vi "Dashboard Main.vi"() -> ()   [LabVIEW 2017]
uses:
  <vilib>/Utility/miscctls.llb/LVRowAndColumnTypeDef.ctl
  <vilib>/event_ctls.llb/eventvkey.ctl
  <vilib>/Rock Robotics/Network Tables/NT Read Numeric Array.vi
  <vilib>/Rock Robotics/WPI/Dashboard/WPI_DashboardLogging Global.vi
panel:
  in  "Camera Settings Right":T1={"Frame Rate"=30, "Compression"=30, "Size"=1, "DB Camera Config"=FALSE} {"Frame Rate" scale=1.0..30.0; "Compression" scale=100.0..-1.0; "Size" items=["640x480", "320x240", "160x120"]}
  in  "Camera Name Right":string(combo)="No Camera Selection"
  out "Camera Info":cluster{"Mbps LED":bool, "Mbps":dbl, "fps":dbl} {"fps" format="%#.1g"; "Mbps" format="%#.1g"}
  in  "Camera Settings":T1={"Frame Rate"=30, "Compression"=30, "Size"=1, "DB Camera Config"=FALSE} {"Frame Rate" scale=1.0..30.0; "Compression" scale=100.0..-1.0; "Size" items=["640x480", "320x240", "160x120"]}
  in  "TCP":refnum<k5>
  in  "Rec Mode":enum32{"Stop", "Record", "Playback"}(radio)
  out "Robot IP":string
  out "Image Message":string="Timeout in Camera Communications"
  in  "Dashboard Tab":T2(tab)
  in  "Select Auto":string(combo)="Select Autonomous ..."
  out "NT Connection":bool
  out "MotorChart R":cluster{"Numeric":dbl, "Numeric":dbl}(graph)
  out "MotorChart L":cluster{"Numeric":dbl, "Numeric":dbl}(graph)
  out "MotorSliders R":cluster{"MotorSlide1":dbl, "MotorSlide2":dbl} {"MotorSlide2" scale=-1.0..1.0 scale format="%#_2e"; "MotorSlide1" scale=-1.0..1.0 scale format="%#_2e"}
  out "MotorSliders L":cluster{"MotorSlide1":dbl, "MotorSlide2":dbl} {"MotorSlide2" scale=-1.0..1.0 scale format="%#_2e"; "MotorSlide1" scale=-1.0..1.0 scale format="%#_2e"}
  out "Gyro":dbl(knob) scale=0.0..360.0
  out "JS1 Z":dbl(slide) scale=-1.0..1.0 scale format="%#_2e"
  out "JS1 Graph":cluster{"X":dbl, "Y":dbl}[](graph)
  out "JS1 Buttons":T3
  out "JS2 Z":dbl(slide) scale=-1.0..1.0 scale format="%#_2e"
  out "JS2 Graph":cluster{"X":dbl, "Y":dbl}[](graph)
  out "JS2 Buttons":T3
  out "Mode":T4(ring)=enum."Auto Disabled"
  out "Camera Image Right":T5(plugin-control)
  in  "DB/String 9":string
  in  "DB/String 8":string
  in  "DB/String 7":string
  in  "DB/String 6":string
  in  "DB/String 5":string
  in  "DB/String 4":string
  in  "DB/String 3":string
  in  "DB/String 2":string
  in  "DB/String 1":string
  in  "DB/String 0":string
  in  "DB/Slider 0":dbl(slide) scale=0.0..5.0
  in  "DB/Slider 1":dbl(slide) scale=0.0..5.0
  in  "DB/Slider 2":dbl(slide) scale=0.0..5.0
  in  "DB/Slider 3":dbl(slide) scale=0.0..5.0
  out "DB/LED 3":bool
  out "DB/LED 2":bool
  out "DB/LED 1":bool
  out "DB/LED 0":bool
  in  "DB/Button 3":bool
  in  "DB/Button 2":bool
  in  "DB/Button 1":bool
  in  "DB/Button 0":bool caption="New Name"
  in  "When Switch on Same Side\nAnd Scale on Wrong Side":u16(ring) items=["Do Nothing"=0, "Cross Auto Line"=4]
  in  "When Switch on Opposite Side\nAnd Scale on Wrong Side":u16(ring) items=["Do Nothing"=0, "Cross AutoLine"=4]
  in  "Direction":u16(ring) items=["Forward (Cube in forks)", "Backward (Cube on shelf)"]
  in  "Starting Position":u16(ring) items=["Left", "Center-Left", "Center", "Center-Right", "Right"]
  in  "When Switch on Opposite Side":u16(ring) items=["Do Nothing"=0, "Cross in Front"=1, "Cross Behind"=2, "Cross Auto Line"=4, "Drive to Null Territory"=5, "Check Scale"=3]
  in  "When Switch on Same Side":u16(ring) items=["Do Nothing"=0, "Proceed"=1, "Drive to Null Territory"=5, "Cross Auto Line"=4, "Check Scale"=3]
  in  "When Switch on Right Side":u16(ring) items=["Do Nothing", "Proceed"]
  in  "When Switch on Left SIde":u16(ring) items=["Do Nothing", "Proceed"]
  in  "Test Slider":dbl(slide) scale=0.0..100.0 scale format="%#_3g"
  in  "On/Off":bool caption="Solenoid"
  in  "Test Name":u16(ring) items=["Select the test to run..."]
  in  "Test Tree":string(tree)
  in  "Motor":cluster{"Value":dbl, "Enable":bool} {"Value" scale=-1.0..1.0 scale format="%#_3g"}
  out "Progress":T6 {"Test Progress" scale=0.0..100.0}
  in  "Rev/Fwd":cluster{"Forward":bool, "Reverse":bool}
  in  "Test Ring":u16(ring) items=["Monochrome", "Color"]
  out "Cmd Status":string
  in  "Execute Command":bool
  in  "Command Params":string[][](table)
  in  "Command Selection":i32(listbox)
  in  "CheckList":i32(listbox)
  out "Tree":string(tree)
  out "Camera Image":T5(plugin-control)
  out "Background":bool
  in  "Camera Name":string(combo)="No Camera Selection"
  # "HW"
  # "HW"
  # "Joysticks"
  # "Drive Motors"
  # "Front"
  # "Right"
  # "Left"
  # "Back"
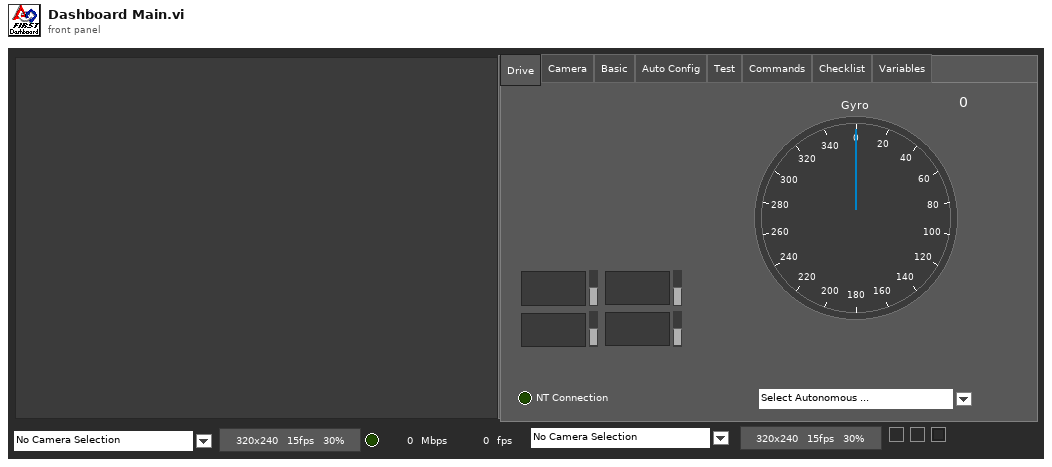
[diagram p1: front panel]
types:
  T1 = cluster{"Frame Rate":i32, "Compression":i32, "Size":u16, "DB Camera Config":bool}
  T2 = enum32{"Drive", "Camera", "Basic", "Auto Config", "Test", "Commands", "Checklist", "Variables"}
  T3 = cluster{bool, bool, bool, bool, bool, bool, bool, bool, bool, bool, bool, bool}
  T4 = enum8{"Tele-Op Disabled", "Tele-Op Enabled", "Auto Disabled", "Auto Enabled", "Test Disabled", "Test Enabled", "Disconnected", "No Code", "E-Stop"}
  T5 = typedef "IMAQ Image.ctl" = refnum<image>
  T6 = cluster{"Test Progress":u8, "Test Progress Text":string}
  T7 = cluster{"Save Path":path, "Interval (s)":dbl, "Keep":i32}
  T8 = enum32{"Drive", "Camera", "Basic", "Custom", "Test", "Commands", "Checklist", "Variables"}
  T9 = typedef "Image Type" = u32
  T10 = cluster{"IDs":cluster{"RPC field ID":u16, "Unique ID":u16}, "String":string}
  T11 = cluster{"Error Strings":string, "Disable Counts":cluster{u16, u16}, "Rail Faults":cluster{u16, u16, u16}, "Robot IP":string, "DB Mode":u8, "Event Info":cluster{"Name":string, "Type":u8, "Number":u16, "Replay":u8}}
  T12 = cluster{"Storage":cluster{"Disk Free":u64, "RAM Block":u32, "RAM free":u32}, "CPU Utilization":cluster{"CPU % ISR":sgl, "CPU % Time Crit":sgl, "CPU % Timed Str":sgl, "CPU % High":sgl, "CPU % Above":sgl, "CPU % Normal":sgl, "CPU % Low":sgl}, "CAN":cluster{"% Bus Utilization":sgl, "Bus Off Cnt":u32, "TX_FIFO Full Cnt":u32, "Receive Error Cnt":u8, "Transmit Error Cnt":u8}, "HID":cluster{"HID Outputs":u32, "Rumble Low":u16, "Rumble High":u16}[]}
  T13 = cluster{"Status bits":cluster{"Test Mode":bool, "Autonomous":bool, "Enabled":bool, "Code Start":bool, "Brownout":bool, "Reserved 2":bool, "Reserved 3":bool, "E-Stop":bool}, "Code Trace":cluster{"Disabled":bool, "TeleOp":bool, "Auto":bool, "Test":bool}, "Controller Type":enum16{"unknown", "cRIO", "roboRio"}, "Code?":enum16{"unknown", "noCode", "code"}, "Battery V":dbl}
  T14 = cluster{"Control Bits":cluster{"TestMode":bool, "Autonomous":bool, "Enabled":bool, "FMS Present":bool, bool, bool, bool, "E-Stop":bool}, "Team Station ":u8, "Countdown":sgl, "Joystick Values":cluster{"Axes":dbl[], "Buttons":bool[], "POVs":i16[]}[]}
  T15 = cluster{"Axes":dbl[], "Buttons":bool[], "POVs":i16[]}[]
  T16 = cluster{"Axes":dbl[], "Buttons":bool[], "POVs":i16[]}
  T17 = cluster{"Buttons[0]":bool, "Buttons[1]":bool, "Buttons[2]":bool, "Buttons[3]":bool, "Buttons[4]":bool, "Buttons[5]":bool, "Buttons[6]":bool, "Buttons[7]":bool, "Buttons[8]":bool, "Buttons[9]":bool, "Buttons[10]":bool, "Buttons[11]":bool}
  T18 = cluster{"Camera Image":refnum<vi>, "Dashboard Tab":refnum<vi>, "Background":refnum<vi>, "Rec Mode":refnum<vi>, "Test Slider":refnum<vi>, "On/Off ":refnum<vi>, "Test Ring":refnum<vi>, "Rev/Fwd":refnum<vi>, "Test Name":refnum<vi>, "Motor":refnum<vi>, "Progress":refnum<vi>, "CheckList":refnum<vi>, "Tree":refnum<vi>, "Test Tree":refnum<vi>, "Command Params":refnum<vi>, "Command Selection":refnum<vi>, "Execute Command":refnum<vi>, "Cmd Status":refnum<vi>, "Camera Settings":refnum<vi>, "Camera Name":refnum<vi>, "Camera Info":refnum<vi>, "Camera Settings Right":refnum<vi>, "Camera Name Right":refnum<vi>, "Camera Image Right":refnum<vi>}
  T19 = cluster{"Camera Name Right":string, string, "Saved DB Images Info":cluster{"Save Path":path, "Interval (s)":dbl, "Keep":i32}}
  T20 = cluster{"Camera Name":string, string, "Saved DB Images Info":cluster{"Save Path":path, "Interval (s)":dbl, "Keep":i32}}
  T21 = cluster{"Operation":enum16{"Update", "Clear"}, "Color Box":u32}[]
  T22 = typedef "eventvkey.ctl" = enum16{"ASCII", "Enter", "Return", "Shift", "Ctrl", "Alt", "Cmd", "Opt", "Caps", "NumLock", "Clear", "Break", "Up", "Down", "Left", "Right", "Insert", "Delete", "Home", "End", "PageUp", "PageDown", "Escape", "Help", "Pause", "ScrollLock", "F1", "F2", "F3", "F4", "F5", "F6", "F7", "F8", "F9", "F10", "F11", "F12", "F13", "F14", "F15", "F16", "F17", "F18", "F19", "F20", "F21", "F22", "F23", "F24", "Play", "VolumeUp", "VolumeDown", "Mute", "Two Byte Char"}
  T23 = cluster{"Image Size":bool, "Image Type":bool, "Pixel Value":bool, "ROI Information":bool, "Zoom Factor":bool}
  T24 = cluster{"Operation":enum16{"Update", "Clear"}, "Color Box":u32}
  T25 = typedef "LVRowAndColumnTypeDef.ctl" = cluster{"Row":i32, "Column":i32}
  T26 = cluster{"Shift":bool, "Ctrl":bool, "Alt":bool, "Cmd":bool, "Opt":bool}
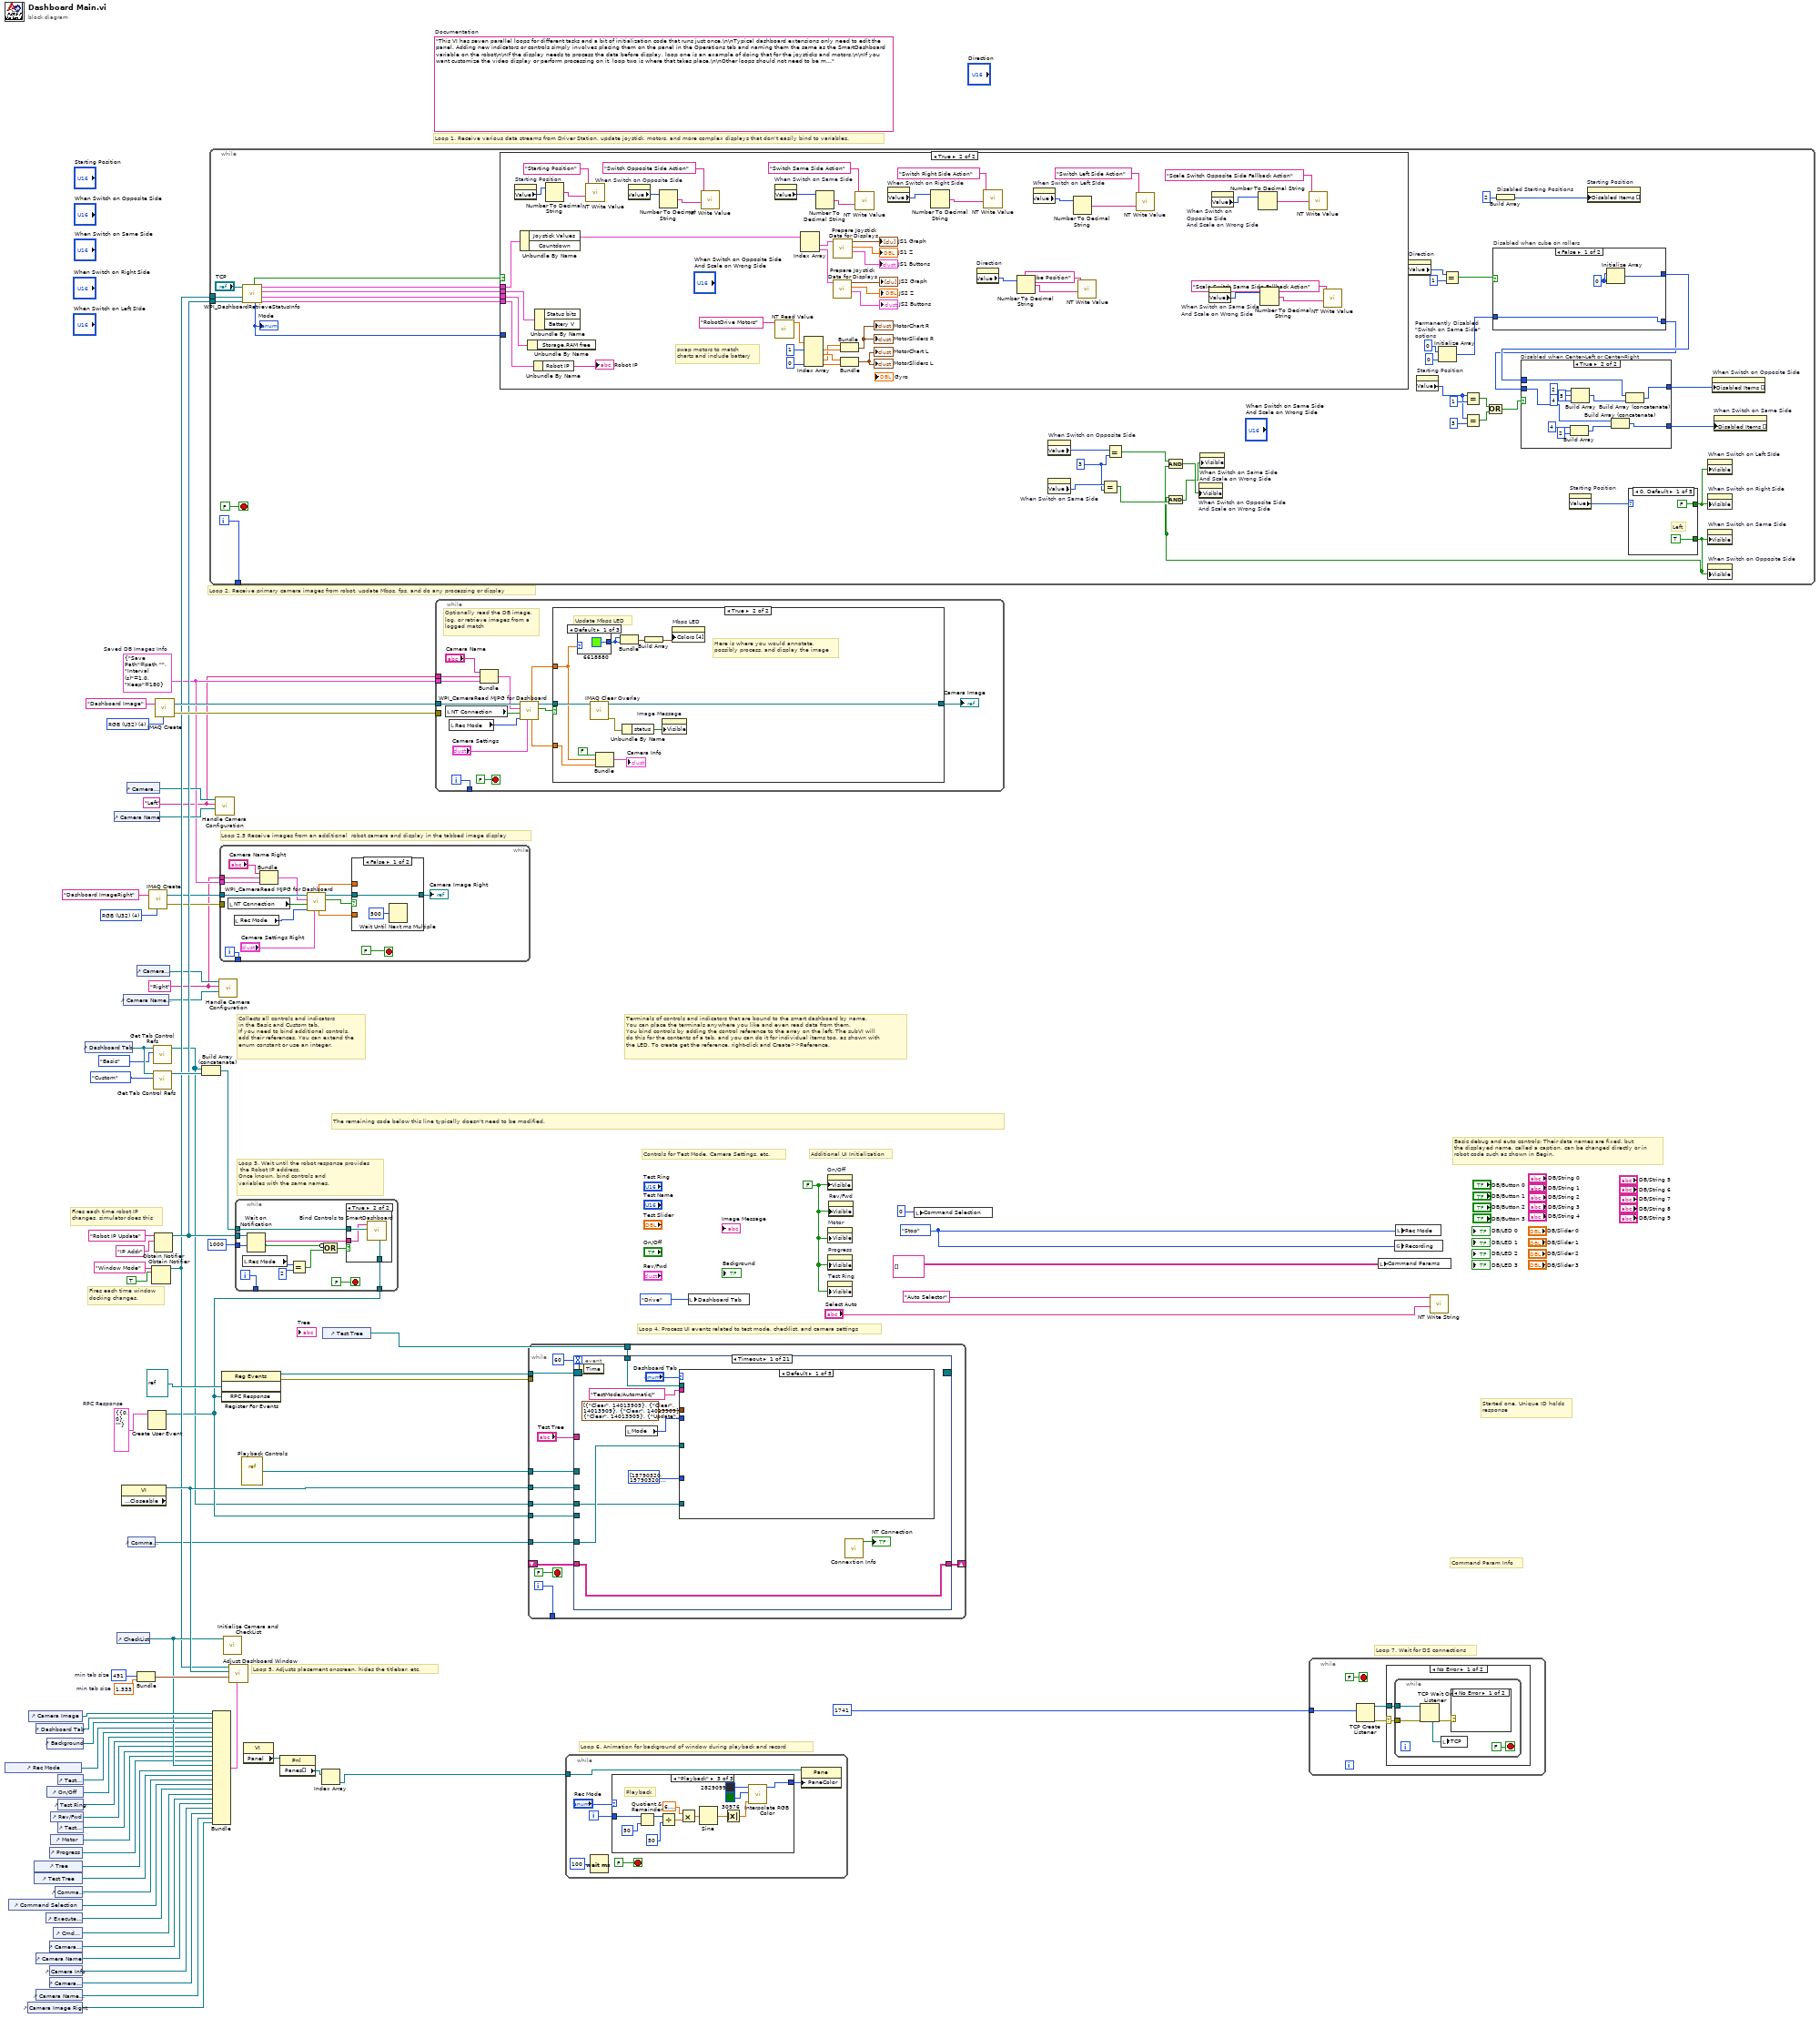
[diagram p0: block diagram]
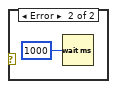
[diagram p3: hidden frame]
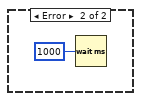
[diagram p4: hidden frame]
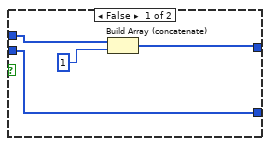
[diagram p5: hidden frame]
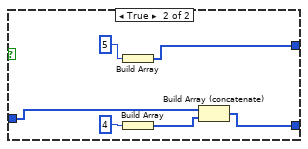
[diagram p6: hidden frame]
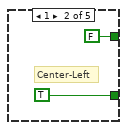
[diagram p7: hidden frame]
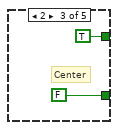
[diagram p8: hidden frame]
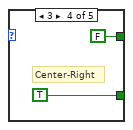
[diagram p9: hidden frame]
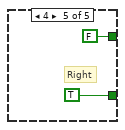
[diagram p10: hidden frame]
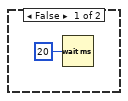
[diagram p11: hidden frame]
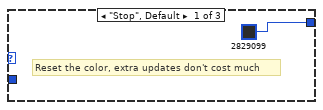
[diagram p12: hidden frame]
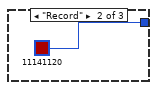
[diagram p13: hidden frame]
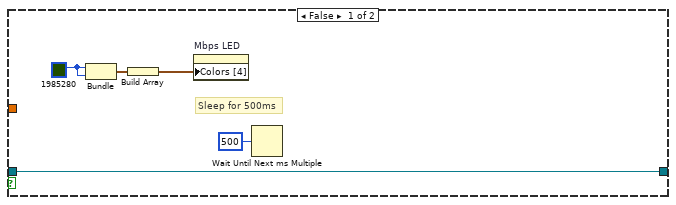
[diagram p15: hidden frame]
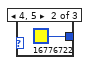
[diagram p16: hidden frame]
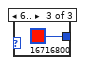
[diagram p17: hidden frame]
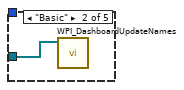
[diagram p18: hidden frame]
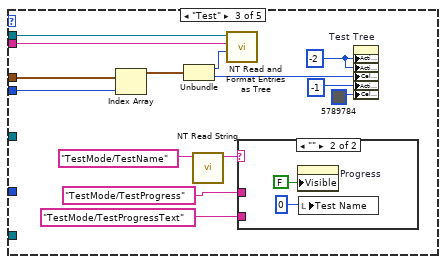
[diagram p19: hidden frame]
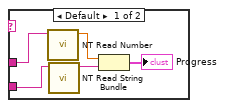
[diagram p20: hidden frame]
diagram:
  w3 = T7 {"Save Path"=path "", "Interval (s)"=1.0, "Keep"=180}  # Saved DB Images Info
  w2 = "Right"
  w1 = "Left"
  w13 = T9 4 items=["Grayscale (U8)", "Grayscale (I16)", "Grayscale (SGL)", "Complex (CSG)", "RGB (U32)", "HSL (U32)", "RGB (U64)"] ("Image Type")
  w29 = T10 {"IDs"={"RPC field ID"=0, "Unique ID"=0}, "String"=""}  # RPC Response
  w52 = 491  # min tab size
  w51 = 1.333  # min tab size
  w59 = enum32{"Stop", "Record", "Playback"}."Stop" ("Rec Mode")
  w36 = FALSE ("Visible")
  (unwired) "This VI has seven parallel loops for different tasks and a bit of initialization code that runs just once.\n\nTypical dashboard extensions only need to edit the panel. Adding new indicators or controls simply involves placing them on the panel in the Operations tab and naming them the same as the SmartDashboard variable on the robot\n\nIf the display needs to process the data before display, loop one is an example of doing that for the joysticks and motors.\n\nIf you want customize the video display or perform processing on it, loop two is where that takes place.\n\nOther loops should not need to be modified. They are pretty standard, and document the task they perform."  # Documentation
  w76 = T9 4 items=["Grayscale (U8)", "Grayscale (I16)", "Grayscale (SGL)", "Complex (CSG)", "RGB (U32)", "HSL (U32)", "RGB (U64)"] ("Image Type")
  # "Loop 2.5 Receive images from an additional  robot camera and display in the tabbed image display"
  # "Command Param Info"
  # "Started one, Unique ID holds\nresponse"
  # "Loop 7. Wait for DS connections"
  # "Basic debug and auto controls: Their data names are fixed, but\nthe displayed name, called a caption, can be changed directly or in\nrobot code such as shown in Begin."
  # "Controls for Test Mode, Camera Settings, etc."
  # "Additional UI Initialization"
  # "Loop 6. Animation for background of window during playback and record"
  # "Fires each time robot IP\nchanges, simulator does this"
  # "Fires each time window\ndocking changes."
  # "Collects all controls and indicators\nin the Basic and Custom tab.\nIf you need to bind additional controls,\nadd their references. You can extend the\nenum constant or use an integer."
  # "The remaining code below this line typically doesn't need to be modified."
  # "Loop 4. Process UI events related to test mode, checklist, and camera settings"
  # "Terminals of controls and indicators that are bound to the smart dashboard by name.\nYou can place the terminals anywhere you like and even read data from them.\nYou bind controls by adding the control reference to the array on the left. The subVI will\ndo this for the contents of a tab, and you can do it for individual items too, as shown with\nthe LED. To create get the reference, right-click and Create>>Reference."
  # "Loop 3. Wait until the robot response provides\n the Robot IP address.\nOnce known, bind controls and\nvariables with the same names."
  # "Loop 5. Adjusts placement onscreen, hides the titlebar, etc."
  # "Loop 1. Receive various data streams from Driver Station, update joystick, motors, and more complex displays that don't easily bind to variables."
  # "Loop 2. Receive primary camera images from robot, update Mbps, fps, and do any processing or display"
  n1 = control-ref of="Rec Mode"() -> (w42:refnum<vi>)
  n2 = control-ref of="Command Selection"() -> (w28:refnum<vi>)
  n3 = control-ref of="Camera Image Right"() -> (w6:refnum<vi>)
  n4 = control-ref of="Camera Image"() -> (w54:refnum<vi>)
  n5 = control-ref of="Tree"() -> (w46:refnum<vi>)
  n6 = control-ref of="Test Tree"() -> (w45:refnum<vi>)
  n7 = control-ref of="Dashboard Tab"() -> (w53:refnum<vi>)
  n8 = control-ref of="Camera Name"() -> (w19:refnum<vi>)
  n9 = control-ref of="Camera Name Right"() -> (w7:refnum<vi>)
  n10 = control-ref of="Execute Command"() -> (w30:refnum<vi>)
  n11 = control-ref of="Background"() -> (w49:refnum<vi>)
  n12 = control-ref of="On/Off"() -> (w40:refnum<vi>)
  n13 = control-ref of="Progress"() -> (w37:refnum<vi>)
  n14 = control-ref of="Camera Settings"() -> (w20:refnum<vi>)
  n15 = control-ref of="Camera Info"() -> (w18:refnum<vi>)
  n16 = control-ref of="Camera Settings Right"() -> (w8:refnum<vi>)
  n17 = control-ref of="Rev/Fwd"() -> (w38:refnum<vi>)
  n18 = control-ref of="Motor"() -> (w43:refnum<vi>)
  n19 = control-ref of="Cmd Status"() -> (w24:refnum<vi>)
  n20 = control-ref of="Command Params"() -> (w31:refnum<vi>)
  n21 = control-ref of="Test Slider"() -> (w41:refnum<vi>)
  n22 = control-ref of="Test Ring"() -> (w39:refnum<vi>)
  n23 = control-ref of="Test Name"() -> (w44:refnum<vi>)
  n24 = control-ref of="Dashboard Tab"() -> (w57:refnum<vi>)
  n25 = control-ref of="Camera Name"() -> (w21:refnum<vi>)
  n26 = control-ref of="CheckList"() -> (w47:refnum<vi>)
  n27 = property class="VI" props=["Front Panel.Closeable"]() -> (reference out=w58:refnum<vi>)  [unwired: 2 in, 2 out]
  n28 = control-ref of="Camera Name Right"() -> (w9:refnum<vi>)
  n29 = control-ref of="Camera Settings"() -> (w22:refnum<vi>)
  n30 = control-ref of="Command Params"() -> (w23:refnum<vi>)
  n31 = control-ref of="Camera Settings Right"() -> (w10:refnum<vi>)
  n32 = Bundle("min tab size"=w52, "min tab size"=w51) -> (w50:cluster{"min tab size":i32, "min tab size":dbl})  [unwired: 1 in]
  n33 = Create User Event(user event datatype=w29) -> (user event=w25:refnum<user-event>)  [unwired: 1 in, 1 out]
  n34 = call "IMAQ Create"("Image Name"="Dashboard ImageRight", "Image Type"=w13) -> ("New Image"=w12:T5, "error out"=w11:errorcluster)  [unwired: 2 in, 1 out]
  n35 = Obtain Notifier(name (unnamed)="Window Mode", notification data type=TRUE) -> (notifier out=w34:refnum<notifier>)  [unwired: 2 in, 2 out]
  n36 = call <vilib>:"Get Tab Control Refs.vi"("Page Index"=T8."Basic" ("Dashboard Tab"), "TabControl in"=w57) -> ("ControlsOnPage"=w17:refnum<vi>[])  [unwired: 9 in]
  n37 = call <vilib>:"Get Tab Control Refs.vi"("Page Index"=T8."Custom" ("Dashboard Tab"), "TabControl in"=w57) -> ("ControlsOnPage"=w56:refnum<vi>[])  [unwired: 9 in]
  n38 = Obtain Notifier(name (unnamed)="Robot IP Update", notification data type="IP Addr" ("name (unnamed)")) -> (notifier out=w35:refnum<notifier>)  [unwired: 2 in, 2 out]
  n39 = call "IMAQ Create"("Image Name"="Dashboard Image", "Image Type"=w76) -> ("New Image"=w74:T5, "error out"=w73:errorcluster)  [unwired: 2 in, 1 out]
  n40 = Build Array (concatenate)(w17, w56) -> (w55:refnum<vi>[])
  n41 = while {
    tunnel: [w114] -> _
    tunnel: w35 -> [w108]
    tunnel: w34 -> [w105]
    i -> [w114]
    stop <- FALSE stop-if-true
    w82 = 3
    n42 = call <vilib>:"WPI_DashboardRetrieveStatusInfo.vi"("Binding Refnum"=w108, "Window Mode Notifier"=w105, "TCP Cnx"="TCP") -> ("Power and Errors"=w109:T11, "Robot Metrics"=w112:T12, "Status Info"=w113:T13, "Control Info"=w110:T14, "Robot Mode"=w107:T4, "Process?"=w111:bool)  [unwired: 3 in]
    "Mode" <- w107
    n43 = case shown="True" w111 {
      tunnel: w113 -> [_ w198]
      tunnel: w112 -> [_ w197]
      tunnel: w110 -> [_ w196]
      tunnel: w109 -> [_ w195]
      tunnel: w107 -> [_ _]
      frame False {
        n44 = Wait (ms)(milliseconds to wait=u32 20) -> ()  [unwired: 1 out]
      }
      frame True {
        # "swap motors to match\ncharts and include battery"
        n45 = property on="Starting Position" class="Ring (strict)"() -> ("Value"=w172:u16)  [unwired: 2 in, 2 out]
        n46 = Unbundle By Name(w196) -> ("Joystick Values"=w186:T15)  [unwired: 1 out]
        n47 = Unbundle By Name(w197) -> ()  [unwired: 1 out]
        n48 = Unbundle By Name(w195) -> ("Robot IP"=→"Robot IP":string)
        n49 = Unbundle By Name(w198) -> ()  [unwired: 2 out]
        n50 = Number To Decimal String(number=w172) -> (decimal integer string=w174:string)  [unwired: 1 in]
        n51 = call-poly <vilib>:"NT Write Value.vi"("String"=w174, "Name"="Starting Position") -> ()  [unwired: 9 in, 1 out]
        n52 = property on="When Switch on Opposite Side" class="Ring (strict)"() -> ("Value"=w171:u16)  [unwired: 2 in, 2 out]
        n53 = Number To Decimal String(number=w171) -> (decimal integer string=w157:string)  [unwired: 1 in]
        n54 = call-poly <vilib>:"NT Write Value.vi"("String"=w157, "Name"="Switch Opposite Side Action") -> ()  [unwired: 9 in, 1 out]
        n55 = property on="When Switch on Same Side" class="Ring (strict)"() -> ("Value"=w170:u16)  [unwired: 2 in, 2 out]
        n56 = call-poly <vilib>:"NT Read Value.vi"("Name"="RobotDrive Motors") -> ("Numeric Array"=w176:dbl[])  [unwired: 9 in, 1 out]
        n57 = Index Array(array=w186) -> (element #1=w185:T16, element #2=w181:T16)  [unwired: 2 in]
        n58 = Index Array(array=w176, index #1=1, index #4=0) -> (element #1=w190:dbl, element #2=w191:dbl, element #3=w189:dbl, element #4=w194:dbl)  [unwired: 2 in]
        n59 = Number To Decimal String(number=w170) -> (decimal integer string=w167:string)  [unwired: 1 in]
        n60 = call "Prepare Joystick Data for Displays.vi"("Joystick Values"=w181) -> ("Buttons"=→"JS2 Buttons":T17, "Z Axis"=→"JS2 Z":dbl, "Cartesian Data"=→"JS2 Graph":cluster{"X axis":dbl, "X axis":dbl}[])  [unwired: 8 in]
        n61 = call "Prepare Joystick Data for Displays.vi"("Joystick Values"=w185) -> ("Buttons"=→"JS1 Buttons":T17, "Z Axis"=→"JS1 Z":dbl, "Cartesian Data"=→"JS1 Graph":cluster{"X axis":dbl, "X axis":dbl}[])  [unwired: 8 in]
        n62 = Bundle("Numeric"=w189, "Numeric"=w190) -> (→"MotorChart R" →"MotorSliders R":cluster{"Numeric":dbl, "Numeric":dbl})  [unwired: 1 in]
        n63 = Bundle("Numeric"=w191, "Numeric"=w194) -> (→"MotorChart L" →"MotorSliders L":cluster{"Numeric":dbl, "Numeric":dbl})  [unwired: 1 in]
        n64 = call-poly <vilib>:"NT Write Value.vi"("String"=w167, "Name"="Switch Same Side Action") -> ()  [unwired: 9 in, 1 out]
        n65 = property on="When Switch on Right Side" class="Ring (strict)"() -> ("Value"=w169:u16)  [unwired: 2 in, 2 out]
        n66 = Number To Decimal String(number=w169) -> (decimal integer string=w166:string)  [unwired: 1 in]
        n67 = property on="Direction" class="Ring (strict)"() -> ("Value"=w160:u16)  [unwired: 2 in, 2 out]
        n68 = call-poly <vilib>:"NT Write Value.vi"("String"=w166, "Name"="Switch Right Side Action") -> ()  [unwired: 9 in, 1 out]
        n69 = Number To Decimal String(number=w160) -> (decimal integer string=w159:string)  [unwired: 1 in]
        n70 = property on="When Switch on Left SIde" class="Ring (strict)"() -> ("Value"=w168:u16)  [unwired: 2 in, 2 out]
        n71 = Number To Decimal String(number=w168) -> (decimal integer string=w165:string)  [unwired: 1 in]
        n72 = call-poly <vilib>:"NT Write Value.vi"("String"=w159, "Name"="Cube Position") -> ()  [unwired: 9 in, 1 out]
        n73 = call-poly <vilib>:"NT Write Value.vi"("String"=w165, "Name"="Switch Left Side Action") -> ()  [unwired: 9 in, 1 out]
        n74 = property on="When Switch on Same Side\nAnd Scale on Wrong Side" class="Ring (strict)"() -> ("Value"=w153:u16)  [unwired: 2 in, 2 out]
        n75 = property on="When Switch on Opposite Side\nAnd Scale on Wrong Side" class="Ring (strict)"() -> ("Value"=w156:u16)  [unwired: 2 in, 2 out]
        n76 = Number To Decimal String(number=w156) -> (decimal integer string=w155:string)  [unwired: 1 in]
        n77 = Number To Decimal String(number=w153) -> (decimal integer string=w152:string)  [unwired: 1 in]
        n78 = call-poly <vilib>:"NT Write Value.vi"("String"=w155, "Name"="Scale Switch Opposite Side Fallback Action") -> ()  [unwired: 9 in, 1 out]
        n79 = call-poly <vilib>:"NT Write Value.vi"("String"=w152, "Name"="Scale Switch Same Side Fallback Action") -> ()  [unwired: 9 in, 1 out]
      }
    }
    n80 = property on="When Switch on Opposite Side" class="Ring (strict)"() -> ("Value"=w84:u16)  [unwired: 2 in, 2 out]
    n81 = property on="When Switch on Same Side" class="Ring (strict)"() -> ("Value"=w83:u16)  [unwired: 2 in, 2 out]
    n82 = Equal?(x=w83, y=w82) -> (x = y?=w80:bool)
    n83 = Equal?(x=w84, y=w82) -> (x = y?=w81:bool)
    n84 = property on="Direction" class="Ring (strict)"() -> ("Value"=w103:u16)  [unwired: 2 in, 2 out]
    n85 = property on="Starting Position" class="Ring (strict)"() -> ("Value"=w93:u16)  [unwired: 2 in, 2 out]
    n86 = Initialize Array "Permanently Disabled \"Switch on Same Side\" options"(0, 0 ("dimension size")) -> (w97:i32[])
    n87 = Equal?(x=w103, y=u16 1) -> (x = y?=w101:bool)
    n88 = Equal?(x=w93, y=u16 1) -> (x = y?=w89:bool)
    n89 = Equal?(x=w93, y=u16 3) -> (x = y?=w91:bool)
    n90 = Or(x=w89, y=w91) -> (x .or. y?=w90:bool)
    n91 = case "Disabled when cube on rollers" shown="False" w101 {
      tunnel: [w132 w134] -> w88
      tunnel: [w133 w135] -> w86
      tunnel: w97 -> [w133 w137]
      frame False {
        w131 = 0 ("dimension size")
        n92 = Initialize Array(w131, w131) -> (w132:i32[])
      }
      frame True {
        n93 = Build Array(5) -> (w134:i32[])
        n94 = Build Array(4) -> (w136:i32[])
        n95 = Build Array (concatenate)(w137, w136) -> (w135:i32[])
      }
    }
    n96 = Build Array "Disabled Starting Positions"(2) -> (w98:i32[])
    n97 = case "Disabled when Center-Left or Center-Right" shown="True" w90 {
      tunnel: w88 -> [w118 w127]
      tunnel: [w117 w126] -> w87
      tunnel: w86 -> [w119 w123]
      tunnel: [w119 w122] -> w85
      frame False {
        n98 = Build Array (concatenate)(w118, 1) -> (w117:i32[])
      }
      frame True {
        n99 = Build Array(4, 2 ("element")) -> (w124:i32[])
        n100 = Build Array(2, 5 ("element"), 4 ("element")) -> (w128:i32[])
        n101 = Build Array (concatenate)(w123, w124) -> (w122:i32[])
        n102 = Build Array (concatenate)(w127, w128) -> (w126:i32[])
      }
    }
    n103 = property on="Starting Position" class="Ring (strict)"() -> ("Value"=w100:u16)  [unwired: 2 in, 2 out]
    n104 = property on="Starting Position" class="Ring (strict)"("Disabled Items []"=w98) -> ()  [unwired: 2 in, 2 out]
    n105 = case shown="0, Default" w100 {
      tunnel: [TRUE TRUE FALSE TRUE TRUE] -> w79
      tunnel: [FALSE FALSE TRUE FALSE FALSE] -> w104
      frame 0, Default {
        # "Left"
      }
      frame 1 {
        # "Center-Left"
      }
      frame 2 {
        # "Center"
      }
      frame 3 {
        # "Center-Right"
      }
      frame 4 {
        # "Right"
      }
    }
    n106 = And(x=w81, y=w79) -> (x .and. y?=w78:bool)
    n107 = And(x=w79, y=w80) -> (x .and. y?=w77:bool)
    n108 = property on="When Switch on Opposite Side\nAnd Scale on Wrong Side" class="Ring (strict)"("Visible"=w78) -> ()  [unwired: 2 in, 2 out]
    n109 = property on="When Switch on Same Side\nAnd Scale on Wrong Side" class="Ring (strict)"("Visible"=w77) -> ()  [unwired: 2 in, 2 out]
    n110 = property on="When Switch on Left SIde" class="Ring (strict)"("Visible"=w104) -> ()  [unwired: 2 in, 2 out]
    n111 = property on="When Switch on Right Side" class="Ring (strict)"("Visible"=w104) -> ()  [unwired: 2 in, 2 out]
    n112 = property on="When Switch on Same Side" class="Ring (strict)"("Visible"=w79) -> ()  [unwired: 2 in, 2 out]
    n113 = property on="When Switch on Opposite Side" class="Ring (strict)"("Visible"=w79) -> ()  [unwired: 2 in, 2 out]
    n114 = property on="When Switch on Opposite Side" class="Ring (strict)"("Disabled Items []"=w87) -> ()  [unwired: 2 in, 2 out]
    n115 = property on="When Switch on Same Side" class="Ring (strict)"("Disabled Items []"=w85) -> ()  [unwired: 2 in, 2 out]
  }
  n116 = Bundle("Camera Image"=w54, "Dashboard Tab"=w53, "Background"=w49, "Rec Mode"=w42, "Test Slider"=w41, "On/Off"=w40, "Test Ring"=w39, "Rev/Fwd"=w38, "Test Name"=w44, "Motor"=w43, "Progress"=w37, "CheckList"=w47, "Tree"=w46, "Test Tree"=w45, "Command Params"=w31, "Command Selection"=w28, "Execute Command"=w30, "Cmd Status"=w24, "Camera Settings"=w20, "Camera Name"=w19, "Camera Info"=w18, "Camera Settings Right"=w8, "Camera Name Right"=w7, "Camera Image Right"=w6) -> (w48:T18)  [unwired: 1 in]
  n117 = call "Handle Camera Configuration.vi"("CameraNameRef"=w21, "Display Name"=w1, "ClusterRef"=w22) -> ()  [unwired: 9 in]
  n118 = call "Handle Camera Configuration.vi"("CameraNameRef"=w9, "Display Name"=w2, "ClusterRef"=w10) -> ()  [unwired: 9 in]
  n119 = while {
    tunnel: w12 -> [w213]
    tunnel: w11 -> [_]
    tunnel: [w208] -> _
    tunnel: w3 -> [w202]
    tunnel: w2 -> [w199]
    i -> [w208]
    stop <- FALSE stop-if-true
    n120 = local read "NT Connection"() -> (w203:bool)
    n121 = local read "Rec Mode"() -> (w212:enum32{"Stop", "Record", "Playback"})
    n122 = Bundle("Camera Name Right"="Camera Name Right", w199, "Saved DB Images Info"=w202) -> (w201:T19)  [unwired: 1 in]
    n123 = call <vilib>:"WPI_CameraRead MJPG for Dashboard.vi"("Camera Settings"="Camera Settings Right", "Rec Mode"=w212, "NT Connection"=w203, "Capture Info"=w201, "Refnum in"=w213) -> ("Active"=w207:bool, "Refnum out"=w210:T5, "FPS"=w205:dbl, "Bandwidth (Mbps)"=w206:dbl)  [unwired: 3 in]
    n124 = case shown="False" w207 {
      tunnel: w210 -> [w214 w216]
      tunnel: w206 -> [_ _]
      tunnel: w205 -> [_ _]
      tunnel: [w214 w216] -> w204
      frame False {
        n125 = Wait Until Next ms Multiple(millisecond multiple=u32 500) -> ()  [unwired: 1 out]
      }
      frame True {
      }
    }
    "Camera Image Right" <- w204
  }
  n126 = register-events(refnum<vi> refnum, w25) -> (reference out=w63:refnum<event-registration>, error out=w62:errorcluster)  [unwired: 2 in]
  n127 = call "Initialize Camera and CheckList.vi"("ListBox in"=w47) -> ()  [unwired: 11 in]
  n128 = call "Adjust Dashboard Window.vi"("Sizing Refnums"=w48, "Size Constraints"=w50, "VI"=w58, "WIn Mode"=w34) -> ()  [unwired: 8 in]
  n129 = while {
    tunnel: w55 -> [w228]
    tunnel: w35 -> [w226]
    tunnel: [w224] -> _
    tunnel: u32 1000 ("milliseconds to wait") -> [w223]
    tunnel: w25 -> [w217]
    i -> [w224]
    stop <- FALSE stop-if-true
    n130 = local read "Rec Mode"() -> (w219:enum32{"Stop", "Record", "Playback"})
    n131 = Wait on Notification(notifier=w226, timeout in ms (-1)=w223) -> (notification=w225:string, timed out?=w221:bool)  [unwired: 2 in, 2 out]
    n132 = Equal?(x=w219, y=u16 2 ("Rec Mode")) -> (x = y?=w220:bool)
    n133 = Compound Arithmetic op=OR(invert w221, w220) -> (w222:bool)
    n134 = case shown="True" w222 {
      tunnel: w228 -> [_ w231]
      tunnel: w225 -> [_ w230]
      tunnel: w217 -> [_ w229]
      frame False {
      }
      frame True {
        n135 = call <vilib>:"Bind Controls to SmartDashboard.vi"("RPC ref"=w229, "Bound Control Refs"=w231, "Server IP Address"=w230) -> ()  [unwired: 9 in]
      }
    }
  }
  n136 = vi-ref "Playback Controls.vi"() -> (w64:refnum<vi>)
  n137 = property class="VI"() -> ("Panel"=w66:refnum<vi>)  [unwired: 2 in, 2 out]
  n138 = property class="Pnl"(reference=w66) -> ("Panes[]"=w67:refnum<vi>[])  [unwired: 1 in, 2 out]
  n139 = Index Array(array=w67) -> (element=w65:refnum<vi>)  [unwired: 1 in]
  n140 = control-ref of="Test Tree"() -> (w68:refnum<vi>)
  n141 = while {
    tunnel: w74 -> [w244]
    tunnel: w73 -> [_]
    tunnel: [w245] -> _
    tunnel: w3 -> [w235]
    tunnel: w1 -> [w232]
    i -> [w245]
    stop <- FALSE stop-if-true
    # "Optionally read the DB image,\nlog, or retrieve images from a\nlogged match"
    n142 = local read "NT Connection"() -> (w236:bool)
    n143 = local read "Rec Mode"() -> (w240:enum32{"Stop", "Record", "Playback"})
    n144 = Bundle("Camera Name"="Camera Name", w232, "Saved DB Images Info"=w235) -> (w234:T20)  [unwired: 1 in]
    n145 = call <vilib>:"WPI_CameraRead MJPG for Dashboard.vi"("Camera Settings"="Camera Settings", "Rec Mode"=w240, "NT Connection"=w236, "Capture Info"=w234, "Refnum in"=w244) -> ("Active"=w242:bool, "Refnum out"=w243:T5, "FPS"=w241:dbl, "Bandwidth (Mbps)"=w239:dbl)  [unwired: 3 in]
    n146 = case shown="True" w242 {
      tunnel: w243 -> [w247 w258]
      tunnel: w239 -> [_ w255]
      tunnel: w241 -> [_ w256]
      tunnel: [w247 w252] -> w237
      frame False {
        w249 = u32 1985280 ("Color Box")
        # "Sleep for 500ms"
        n147 = Bundle("Color Box"=w249, "Color Box"=w249) -> (w250:cluster{"Color Box":u32, "Color Box":u32})  [unwired: 1 out]
        n148 = Build Array(w250) -> (w248:cluster{"Color Box":u32, "Color Box":u32}[])
        n149 = property on="Mbps LED" class="Bool (strict)"("Colors [4]"=w248) -> ()  [unwired: 2 in, 2 out]
        n150 = Wait Until Next ms Multiple(millisecond multiple=u32 500) -> ()  [unwired: 1 out]
      }
      frame True {
        # "Here is where you would annotate,\npossibly process, and display the image"
        # "Update Mbps LED"
        n151 = case shown="Default" w255 {
          tunnel: [u32 6618880 ("Color Box") u32 16776722 ("Color Box") u32 16716800 ("Color Box")] -> w259
          frame Default {
          }
          frame 4, 5 {
          }
          frame 6.. {
          }
        }
        n152 = call "IMAQ Clear Overlay"("Image"=w258) -> ("error out"=w261:errorcluster, "Image Out"=w252:T5)  [unwired: 2 in, 7 out]
        n153 = Bundle(FALSE, "Bandwidth (Mbps)"=w255, "FPS"=w256) -> (→"Camera Info":cluster{bool, "Bandwidth (Mbps)":dbl, "FPS":dbl})  [unwired: 1 in]
        n154 = Bundle("Color Box"=w259, "Color Box"=w259) -> (w260:cluster{"Color Box":u32, "Color Box":u32})  [unwired: 1 out]
        n155 = Unbundle By Name(w261) -> ("status"=w262:bool)
        n156 = Build Array(w260) -> (w257:cluster{"Color Box":u32, "Color Box":u32}[])
        n157 = property on="Image Message" class="Str"("Visible"=w262) -> ()  [unwired: 2 in, 2 out]
        n158 = property on="Mbps LED" class="Bool (strict)"("Colors [4]"=w257) -> ()  [unwired: 2 in, 2 out]
      }
    }
    "Camera Image" <- w237
  }
  n159 = while {
    tunnel: [w275] -> _
    tunnel: w68 -> [w274]
    tunnel: w64 -> [w273]
    tunnel: w63 -> [w272]
    tunnel: w62 -> [_]
    tunnel: w58 -> [w271]
    tunnel: w25 -> [w270]
    tunnel: w23 -> [w269]
    shift-right: [w268] -> _
    shift-left: _ -> [w267]
    tunnel: w17 -> [w266]
    i -> [w275]
    stop <- FALSE stop-if-true
    n160 = event shown="[0] Timeout" {
      selector: w272 -> [_ _ _ _ _ _ _ _ _ _ _ _ _ _ _ _ _ _ _ _ _]
      dyn-events: [_ _ _ _ _ _ _ _ _ _ _ _ _ _ _ _ w535 _ _ _ _] -> _
      timeout: u32 60 ("milliseconds to wait") -> [_ _ _ _ _ _ _ _ _ _ _ _ _ _ _ _ _ _ _ _ _]
      tunnel: w274 -> [w287 _ _ _ _ _ _ _ _ _ _ _ _ _ _ _ _ _ _ _ _]
      tunnel: "Test Tree" -> [_ _ _ _ _ _ _ _ _ _ _ w502 w510 w512 w516 w524 _ _ _ _ _]
      tunnel: w273 -> [_ _ _ _ _ _ _ _ _ _ _ _ _ _ _ _ w537 _ w555 _ _]
      tunnel: w271 -> [_ _ _ _ _ _ _ _ _ _ _ _ _ _ _ _ w533 _ _ _ _]
      tunnel: w270 -> [_ _ _ _ _ _ _ _ _ _ _ _ _ _ _ _ w531 _ _ _ _]
      tunnel: w269 -> [w282 _ _ _ _ _ w453 _ _ _ _ _ _ _ _ _ _ _ _ _ _]
      tunnel: [w281 w330 w432 w437 w446 w450 w451 w460 w470 w477 w489 w501 w508 w511 w515 w523 w530 w550 w552 w556 w569] -> w268
      tunnel: w267 -> [w281 w330 w432 w437 w446 w450 w451 _ _ w477 w489 w501 w508 w511 w515 w523 w530 w550 w552 w556 w569]
      tunnel: w266 -> [w279 _ _ _ _ _ _ _ _ _ _ _ _ _ _ _ _ _ _ _ _]
      event Timeout {
        n161 = event-data() -> ()  [unwired: 1 in, 1 out]
        n162 = local read "Mode"() -> (w284:T4)
        n163 = case shown="Default" "Dashboard Tab" {
          tunnel: w287 -> [_ _ w303 _ _]
          tunnel: "TestMode/Automatic/" ("Name Pattern") -> [_ _ w302 _ _]
          tunnel: T21 [{"Operation"=enum."Clear", "Color Box"=14013909}, {"Operation"=enum."Clear", "Color Box"=14013909}, {"Operation"=enum."Clear", "Color Box"=14013909}, {"Operation"=enum."Clear", "Color Box"=14013909}, {"Operation"=enum."Update", "Color Box"=14013909}, {"Operation"=enum."Update", "Color Box"=16777215}, {"Operation"=enum."Clear", "Color Box"=14013909}, {"Operation"=enum."Clear", "Color Box"=14013909}, {"Operation"=enum."Clear", "Color Box"=14013909}] -> [_ _ w295 _ w323]
          tunnel: w284 -> [_ _ w294 _ w322]
          tunnel: u32[] [15790320, 15790320, 15790320, 15790320, 16777215, 16777215, 15790320, 15790320, 15790320] -> [_ _ _ _ w328]
          tunnel: w282 -> [_ _ _ _ w316]
          tunnel: w279 -> [_ w289 _ _ _]
          frame Default {
          }
          frame "Basic" {
            n164 = call <vilib>:"WPI_DashboardUpdateNames.vi"("Controls on Tab"=w289) -> ()  [unwired: 11 in]
          }
          frame "Test" {
            w301 = -2 ("Active Item:Row Number")
            n165 = Index Array(array=w295, index=w294) -> (element=w296:T24)
            n166 = Unbundle(w296) -> ("Operation"=w297:enum16{"Update", "Clear"}, "Color Box"=w298:u32)
            n167 = call <vilib>:"NT Read String.vi"("Name"="TestMode/TestName") -> ("String"=w292:string)  [unwired: 9 in, 1 out]
            n168 = call <vilib>:"NT Read and Format Entries as Tree.vi"("Operation"=w297, "Name Pattern"=w302, "Tree Refnum"=w303) -> ()  [unwired: 7 in, 2 out]
            n169 = case shown="\"\"" w292 {
              tunnel: "TestMode/TestProgress" ("Name") -> [w305 _]
              tunnel: "TestMode/TestProgressText" ("Name") -> [w304 _]
              frame Default {
                n170 = call <vilib>:"NT Read Number.vi"("Name"=w305) -> ("Numeric"=w306:dbl)  [unwired: 9 in, 1 out]
                n171 = call <vilib>:"NT Read String.vi"("Name"=w304) -> ("String"=w307:string)  [unwired: 9 in, 1 out]
                n172 = Bundle("Numeric"=w306, "String"=w307) -> (→"Progress":cluster{"Numeric":dbl, "String":string})  [unwired: 1 in]
              }
              frame "" {
                n173 = property on="Progress" class="Clust (strict)"("Visible"=FALSE) -> ()  [unwired: 2 in, 2 out]
                n174 = local write "Test Name"(u16 0) -> ()
              }
            }
            n175 = property on="Test Tree" class="Tree (strict)"("Active Item Row Number"=w301, "ActiveColNum"=w301, "CellBG"=w298, "Active Item Row Number"=-1 ("Active Item:Row Number"), "CellBG"=u32 5789784 ("Color Box")) -> ()  [unwired: 2 in, 2 out]
          }
          frame "Variables" {
            w313 = string[] ["CameraPublisher", "Usage", "DB"]  # Items to initially close
            n176 = First Call?() -> (First Call?: T/F=w314:bool)
            n177 = control-ref of="Tree"() -> (w315:refnum<vi>)
            n178 = Select(t=w313, s=w314, f=string[] []) -> (s? t:f=w311:string[])
            n179 = call <vilib>:"NT Read and Format Entries as Tree.vi"("Tags to  Close"=w311, "Tree Refnum"=w315) -> ()  [unwired: 8 in, 2 out]
          }
          frame "Commands" {
            w324 = u32 5789784 ("Color Box")
            w325 = T25 {"Row"=-1, "Column"=-2} ("Active Cell:Active Cell")
            w327 = T25 {"Row"=-2, "Column"=-2} ("Active Cell:Active Cell")
            n180 = Index Array(array=w328, index=w322) -> (element=w326:u32)
            n181 = Index Array(array=w323, index=w322) -> (element=w321:T24)
            n182 = Unbundle(w321) -> ("Operation"=w320:enum16{"Update", "Clear"})  [unwired: 1 out]
            n183 = local read "Command Selection"() -> (w319:i32)
            n184 = property on="Command Selection" class="MCListbox (strict)"("ActiveCell"=w327, "CellBG"=w326, "ActiveCell"=w325, "CellBG"=w324) -> ()  [unwired: 2 in, 2 out]
            n185 = call <vilib>:"WPI_DashboardUpdate RPC Info.vi"("Operation"=w320) -> ("update"=w318:bool, "commands"=w317:string[][])  [unwired: 9 in]
            n186 = property on="Command Selection" class="MCListbox (strict)"("ItemNames"=w317) -> ()  [unwired: 2 in, 2 out]
            n187 = property on="Command Params" class="Tbl (strict)"("Active Cell"=w327, "Cell BG Color"=w326, "Active Cell"=w325, "Cell BG Color"=w324) -> ()  [unwired: 2 in, 2 out]
            n188 = call <vilib>:"WPI_DashboardUpdate Command Params.vi"("Update"=w318, "NewVal"=w319, "Commands"=w317, "Param Tbl"=w316) -> ()  [unwired: 7 in, 1 out]
          }
        }
        n189 = call <vilib>:"Connextion Info.vi"() -> ("Connected"=→"NT Connection":bool)  [unwired: 10 in, 1 out]
      }
      event "Test Tree": Value Change {
        # "Show appropriate\ncontrols"
        n190 = event-data() -> ("CtlRef"=w333:refnum<vi>, "NewVal"=w331:string)  [unwired: 1 in]
        n191 = call <vilib>:"WPI_UtilitiesGetTreeIOName.vi"("NewVal"=w331, "TreeControl in"=w333) -> ("I/O Name"=w334:string)  [unwired: 9 in]
        n192 = case shown="\"Camera\"" w334 {
          selector: w334 -> [_ w341 _ w363 w372 _]
          tunnel: w331 -> [_ _ w360 w362 _ w379]
          tunnel: cluster{string[]}[] [{["640x480", "320x240", "160x120"]}, {["Auto", "Fixed indoor", "Fixed outdoor 1", "Fixed outdoor 2", "Fixed fluorescent 1", "Fixed fluorescent 2", "Hold current"]}, {["Auto", "Flicker-free 50 Hz", "Flicker-free 60 Hz", "Hold current"]}, {["None", "Prioritize frame rate", "Prioritize image quality"]}, {["Monochrome", "Color"]}] -> [_ _ _ _ _ w378]
          frame Default {
            w336 = FALSE ("Visible")
            w335 = FALSE ("Visible")
            n193 = property on="Motor" class="Clust (strict)"("Visible"=w335) -> ()  [unwired: 2 in, 2 out]
            n194 = property on="Test Ring" class="Ring (strict)"("Visible"=w335) -> ()  [unwired: 2 in, 2 out]
            n195 = property on="Rev/Fwd" class="Clust (strict)"("Visible"=w336) -> ()  [unwired: 2 in, 2 out]
            n196 = property on="On/Off" class="Bool (strict)"("Visible"=w336) -> ()  [unwired: 2 in, 2 out]
            n197 = property on="Test Slider" class="Slide (strict)"("Visible"=w336) -> ()  [unwired: 2 in, 2 out]
          }
          frame "Analog Out", "Motor", "PWM" {
            w342 = FALSE ("Visible")
            n198 = case shown="\"Analog Out\"" w341 {
              tunnel: [1.0 ("Value") -1.0 ("Value") 0.0 ("Value")] -> w340
              tunnel: [255.0 ("Value") 1.0 ("Value") 5.0 ("Value")] -> w339
              tunnel: [128.0 ("Value") 0.0 ("Value") 0.0 ("Value")] -> w338
              tunnel: [64.0 ("Value") 0.5 ("Value") 1.0 ("Value")] -> w337
              frame "PWM" {
              }
              frame "Motor", Default {
              }
              frame "Analog Out" {
              }
            }
            n199 = property on="Motor" class="Clust (strict)"("Visible"=TRUE) -> ()  [unwired: 2 in, 2 out]
            n200 = property on="Value" class="Slide (strict)"("Value"=w338, "Scale.Minimum"=w340, "Scale.Maximum"=w339, "Scale.Increment"=w337) -> ()  [unwired: 2 in, 2 out]
            n201 = property on="On/Off" class="Bool (strict)"("Visible"=w342) -> ()  [unwired: 2 in, 2 out]
            n202 = property on="Test Slider" class="Slide (strict)"("Visible"=w342) -> ()  [unwired: 2 in, 2 out]
            n203 = property on="Test Ring" class="Ring (strict)"("Visible"=w342) -> ()  [unwired: 2 in, 2 out]
            n204 = property on="Rev/Fwd" class="Clust (strict)"("Visible"=w342) -> ()  [unwired: 2 in, 2 out]
          }
          frame "Servo" {
            w358 = FALSE ("Visible")
            n205 = call <vilib>:"NT Read Number.vi"("Name"=w360) -> ("Numeric"=w359:dbl)  [unwired: 9 in, 1 out]
            n206 = property on="Test Slider" class="Slide (strict)"("Visible"=TRUE, "Scale.Maximum"=170.0 ("Scale.Range:Maximum")) -> ()  [unwired: 2 in, 2 out]
            n207 = local write "Test Slider"(w359) -> ()
            n208 = property on="Motor" class="Clust (strict)"("Visible"=w358) -> ()  [unwired: 2 in, 2 out]
            n209 = property on="Rev/Fwd" class="Clust (strict)"("Visible"=w358) -> ()  [unwired: 2 in, 2 out]
            n210 = property on="On/Off" class="Bool (strict)"("Visible"=w358) -> ()  [unwired: 2 in, 2 out]
            n211 = property on="Test Ring" class="Ring (strict)"("Visible"=w358) -> ()  [unwired: 2 in, 2 out]
          }
          frame "Relay", "Solenoid" {
            w361 = FALSE ("Visible")
            n212 = property on="Motor" class="Clust (strict)"("Visible"=w361) -> ()  [unwired: 2 in, 2 out]
            n213 = property on="Test Slider" class="Slide (strict)"("Visible"=w361) -> ()  [unwired: 2 in, 2 out]
            n214 = Search and Replace String(input string=w362, search string="/Value  **", replace string="/Direction") -> (result string=w368:string)  [unwired: 5 in, 3 out]
            n215 = property on="Test Ring" class="Ring (strict)"("Visible"=w361) -> ()  [unwired: 2 in, 2 out]
            n216 = call <vilib>:"NT Read String.vi"("Name"=w368) -> ("String"=w366:string)  [unwired: 9 in, 1 out]
            n217 = Equal?(x="Both directions", y=w366) -> (x = y?=w364:bool)
            n218 = Not(x=w364) -> (.not. x?=w365:bool)
            n219 = property on="Rev/Fwd" class="Clust (strict)"("Visible"=w364) -> ()  [unwired: 2 in, 2 out]
            n220 = property on="On/Off" class="Bool (strict)"("Visible"=w365, "Caption.Text"=w363) -> ()  [unwired: 2 in, 2 out]
          }
          frame "Compressor", "Digital Out" {
            w371 = FALSE ("Visible")
            # "Get direction and finish"
            n221 = property on="Motor" class="Clust (strict)"("Visible"=w371) -> ()  [unwired: 2 in, 2 out]
            n222 = property on="Test Slider" class="Slide (strict)"("Visible"=w371) -> ()  [unwired: 2 in, 2 out]
            n223 = property on="Test Ring" class="Ring (strict)"("Visible"=w371) -> ()  [unwired: 2 in, 2 out]
            n224 = property on="On/Off" class="Bool (strict)"("Visible"=TRUE, "Caption.Text"=w372) -> ()  [unwired: 2 in, 2 out]
            n225 = property on="Rev/Fwd" class="Clust (strict)"("Visible"=FALSE) -> ()  [unwired: 2 in, 2 out]
          }
          frame "Camera" {
            n226 = call <vilib>:"Get Last Path Segment.vi"("String in"=w379) -> ("String out"=w380:string)  [unwired: 10 in]
            n227 = property on="On/Off" class="Bool (strict)"("Visible"=FALSE) -> ()  [unwired: 2 in, 2 out]
            n228 = property on="Motor" class="Clust (strict)"("Visible"=FALSE) -> ()  [unwired: 2 in, 2 out]
            n229 = property on="Rev/Fwd" class="Clust (strict)"("Visible"=FALSE) -> ()  [unwired: 2 in, 2 out]
            n230 = case shown="\"White Balance  **\"" w380 {
              tunnel: w379 -> [w386 w395 w404 w413 w422 _ w428]
              tunnel: w378 -> [w384 w392 w401 w410 w419 _ _]
              frame "Size  **" {
                n231 = Index Array(array=w384) -> (element=w383:cluster{string[]})  [unwired: 1 in]
                n232 = call <vilib>:"NT Read String.vi"("Name"=w386) -> ("String"=w385:string)  [unwired: 9 in, 1 out]
                n233 = Unbundle(w383) -> (w381:string[])
                n234 = Match First String(2:w381, 3:w385) -> (0:w382:i32)  [unwired: 1 out]
                n235 = property on="Test Ring" class="Ring (strict)"("Value"=w382, "Strings []"=w381) -> ()  [unwired: 2 in, 2 out]
                n236 = property on="Test Ring" class="Ring (strict)"("Visible"=TRUE) -> ()  [unwired: 2 in, 2 out]
                n237 = property on="Test Slider" class="Slide (strict)"("Visible"=FALSE) -> ()  [unwired: 2 in, 2 out]
              }
              frame "White Balance  **" {
                n238 = Index Array(array=w392, index=1) -> (element=w393:cluster{string[]})
                n239 = call <vilib>:"NT Read String.vi"("Name"=w395) -> ("String"=w394:string)  [unwired: 9 in, 1 out]
                n240 = Unbundle(w393) -> (w390:string[])
                n241 = Match First String(2:w390, 3:w394) -> (0:w389:i32)  [unwired: 1 out]
                n242 = property on="Test Ring" class="Ring (strict)"("Value"=w389, "Strings []"=w390) -> ()  [unwired: 2 in, 2 out]
                n243 = property on="Test Ring" class="Ring (strict)"("Visible"=TRUE) -> ()  [unwired: 2 in, 2 out]
                n244 = property on="Test Slider" class="Slide (strict)"("Visible"=FALSE) -> ()  [unwired: 2 in, 2 out]
              }
              frame "Exposure  **" {
                n245 = Index Array(array=w401, index=2) -> (element=w402:cluster{string[]})
                n246 = call <vilib>:"NT Read String.vi"("Name"=w404) -> ("String"=w403:string)  [unwired: 9 in, 1 out]
                n247 = Unbundle(w402) -> (w398:string[])
                n248 = Match First String(2:w398, 3:w403) -> (0:w399:i32)  [unwired: 1 out]
                n249 = property on="Test Ring" class="Ring (strict)"("Value"=w399, "Strings []"=w398) -> ()  [unwired: 2 in, 2 out]
                n250 = property on="Test Ring" class="Ring (strict)"("Visible"=TRUE) -> ()  [unwired: 2 in, 2 out]
                n251 = property on="Test Slider" class="Slide (strict)"("Visible"=FALSE) -> ()  [unwired: 2 in, 2 out]
              }
              frame "Exposure Priority  **" {
                n252 = Index Array(array=w410, index=3) -> (element=w411:cluster{string[]})
                n253 = call <vilib>:"NT Read String.vi"("Name"=w413) -> ("String"=w412:string)  [unwired: 9 in, 1 out]
                n254 = Unbundle(w411) -> (w407:string[])
                n255 = Match First String(2:w407, 3:w412) -> (0:w408:i32)  [unwired: 1 out]
                n256 = property on="Test Ring" class="Ring (strict)"("Value"=w408, "Strings []"=w407) -> ()  [unwired: 2 in, 2 out]
                n257 = property on="Test Ring" class="Ring (strict)"("Visible"=TRUE) -> ()  [unwired: 2 in, 2 out]
                n258 = property on="Test Slider" class="Slide (strict)"("Visible"=FALSE) -> ()  [unwired: 2 in, 2 out]
              }
              frame "Color Enable  **" {
                n259 = Index Array(array=w419, index=4) -> (element=w420:cluster{string[]})
                n260 = call <vilib>:"NT Read String.vi"("Name"=w422) -> ("String"=w421:string)  [unwired: 9 in, 1 out]
                n261 = Unbundle(w420) -> (w416:string[])
                n262 = Match First String(2:w416, 3:w421) -> (0:w417:i32)  [unwired: 1 out]
                n263 = property on="Test Ring" class="Ring (strict)"("Value"=w417, "Strings []"=w416) -> ()  [unwired: 2 in, 2 out]
                n264 = property on="Test Ring" class="Ring (strict)"("Visible"=TRUE) -> ()  [unwired: 2 in, 2 out]
                n265 = property on="Test Slider" class="Slide (strict)"("Visible"=FALSE) -> ()  [unwired: 2 in, 2 out]
              }
              frame Default {
                n266 = property on="Test Ring" class="Ring (strict)"("Visible"=FALSE) -> ()  [unwired: 2 in, 2 out]
                n267 = property on="Test Slider" class="Slide (strict)"("Visible"=FALSE) -> ()  [unwired: 2 in, 2 out]
              }
              frame "Brightness  **", "Color Level  **", "Compression  **", "FPS  **", "Sharpness  **" {
                n268 = call <vilib>:"NT Read Number.vi"("Name"=w428) -> ("Numeric"=w427:dbl)  [unwired: 9 in, 1 out]
                n269 = local write "Test Slider"(w427) -> ()
                n270 = property on="Test Slider" class="Slide (strict)"("Visible"=TRUE, "Scale.Maximum"=100.0 ("Scale.Range:Maximum")) -> ()  [unwired: 2 in, 2 out]
                n271 = property on="Test Ring" class="Ring (strict)"("Visible"=FALSE) -> ()  [unwired: 2 in, 2 out]
              }
            }
          }
        }
        n272 = property on="Progress" class="Clust (strict)"("Visible"=FALSE) -> ()  [unwired: 2 in, 2 out]
      }
      event "Test Name": Mouse Enter {
        # "Populate the ring with the list of tests"
        n273 = event-data() -> ()  [unwired: 1 in, 1 out]
        n274 = call <vilib>:"NT Read String Array.vi"("Name"="TestMode/TestList") -> ("String Array"=w436:string[])  [unwired: 9 in, 1 out]
        n275 = Build Array (concatenate)("Select the test to run...", w436) -> (w435:string[])
        n276 = property on="Test Name" class="Ring (strict)"("Strings []"=w435) -> ()  [unwired: 2 in, 2 out]
      }
      event "Test Name": Value Change {
        w438 = FALSE ("Visible")
        # "Tell the robot the test name to run"
        n277 = event-data() -> ("NewVal"=w442:u16)  [unwired: 1 in]
        n278 = property on="Test Name" class="Ring (strict)"() -> ("Strings []"=w443:string[])  [unwired: 2 in, 2 out]
        n279 = local write "Progress"(T6 {"Test Progress"=0, "Test Progress Text"=""} ("Progress")) -> ()
        n280 = Index Array(array=w443, index=w442) -> (element=w441:string)
        n281 = call <vilib>:"NT Write String.vi"("String"=w441, "Name"="TestMode/TestName") -> ()  [unwired: 9 in, 1 out]
        n282 = property on="Progress" class="Clust (strict)"("Visible"=TRUE) -> ()  [unwired: 2 in, 2 out]
        n283 = property on="Motor" class="Clust (strict)"("Visible"=w438) -> ()  [unwired: 2 in, 2 out]
        n284 = property on="Test Slider" class="Slide (strict)"("Visible"=w438) -> ()  [unwired: 2 in, 2 out]
        n285 = property on="On/Off" class="Bool (strict)"("Visible"=w438) -> ()  [unwired: 2 in, 2 out]
        n286 = property on="Rev/Fwd" class="Clust (strict)"("Visible"=w438) -> ()  [unwired: 2 in, 2 out]
        n287 = property on="Test Ring" class="Ring (strict)"("Visible"=w438) -> ()  [unwired: 2 in, 2 out]
      }
      event "Select Auto": Mouse Enter {
        # "Populate the combo box with the list of autonomous options"
        n288 = event-data() -> ()  [unwired: 1 in, 1 out]
        n289 = call <vilib>:"NT Read String Array.vi"("Name"="Auto List") -> ("String Array"=w445:string[])  [unwired: 9 in, 1 out]
        n290 = property on="Select Auto" class="CmbBox"("Strings[]"=w445) -> ()  [unwired: 2 in, 2 out]
      }
      event "Select Auto": Value Change {
        # "User modified the Auto Selection. Write to NT variable so robot knows."
        n291 = event-data() -> ("NewVal"=w448:string)  [unwired: 1 in]
        n292 = call <vilib>:"NT Write String.vi"("String"=w448, "Name"="Auto Selector") -> ()  [unwired: 9 in, 1 out]
      }
      event "Command Selection": Value Change {
        # "Get the params and show in table"
        n293 = event-data() -> ("NewVal"=w454:i32)  [unwired: 1 in]
        n294 = property on="Command Selection" class="MCListbox (strict)"() -> ("ItemNames"=w452:string[][])  [unwired: 2 in, 2 out]
        n295 = call <vilib>:"WPI_DashboardUpdate Command Params.vi"("NewVal"=w454, "Commands"=w452, "Param Tbl"=w453) -> ()  [unwired: 8 in, 1 out]
      }
      event "Execute Command": Value Change {
        # "Started one, Unique ID holds\nresponse"
        n296 = event-data() -> ()  [unwired: 1 in, 1 out]
        n297 = property on="Command Selection" class="MCListbox (strict)"() -> ("ItemNames"=w465:string[][])  [unwired: 2 in, 2 out]
        n298 = Index Array(array=w465, index (row)="Command Selection", index (col)=0) -> (element=w463:string)
        n299 = call <vilib>:"Invoke Commands.vi"("Command Params"="Command Params", "Function Name"=w463) -> ("Params"=w459:u8, "Started"=w458:bool)  [unwired: 7 in, 1 out]
        n300 = Array Subset(array="Command Params", length (row)=w459) -> (w460:string[][])  [unwired: 3 in]
        n301 = Select(t="Executing" ("Cmd Status"), s=w458, f="" ("Cmd Status")) -> (s? t:f=→"Cmd Status":string)
      }
      event "Command Selection": Double Click {
        n302 = event-data() -> ("Row"=w473:i32)  [unwired: 1 in]
        n303 = property on="Command Selection" class="MCListbox (strict)"() -> ("ItemNames"=w476:string[][])  [unwired: 2 in, 2 out]
        n304 = local read "Command Params"() -> (w472:string[][])
        n305 = Index Array(array=w476, index (row)=w473, index (col)=0) -> (element=w474:string)
        n306 = call <vilib>:"Invoke Commands.vi"("Command Params"=w472, "Function Name"=w474) -> ("Params"=w471:u8, "Started"=w466:bool)  [unwired: 7 in, 1 out]
        n307 = Array Subset(array=w472, length (row)=w471) -> (w470:string[][])  [unwired: 3 in]
        n308 = Select(t="Executing" ("Cmd Status"), s=w466, f="" ("Cmd Status")) -> (s? t:f=w467:string)
        n309 = local write "Cmd Status"(w467) -> ()
      }
      event "CheckList": Double Click {
        # "Shift clears all"
        # "Update symbols on the listbox"
        n310 = event-data() -> ("PlatMods.Shift"=w478:bool, "Row"=w480:i32)  [unwired: 1 in]
        n311 = case shown="True" w478 {
          tunnel: w480 -> [w484 _]
          tunnel: 1 -> [w483 _]
          frame False {
            n312 = property on="CheckList" class="LstBox (strict)"() -> ("Item Symbols"=w482:i32[])  [unwired: 2 in, 2 out]
            n313 = Replace Array Subset(array=w482, new element=w483, index=w484) -> (w481:i32[])
            n314 = property on="CheckList" class="LstBox (strict)"("Item Symbols"=w481) -> ()  [unwired: 2 in, 2 out]
          }
          frame True {
            w485 = 0 ("Top Row")
            n315 = property on="CheckList" class="LstBox (strict)"() -> ("Number of Rows"=w487:u32)  [unwired: 2 in, 2 out]
            n316 = Initialize Array(0, w487) -> (w486:i32[])
            n317 = property on="CheckList" class="LstBox (strict)"("Top Row"=w485, "Value"=w485, "Item Symbols"=w486) -> ()  [unwired: 2 in, 2 out]
          }
        }
      }
      event "CheckList": Key Down {
        # "Update symbols on the listbox\nLeft and right keys check and uncheck"
        n318 = event-data() -> ("VKey"=w491:T22)  [unwired: 1 in]
        n319 = case shown="\"Left\", \"Right\"" w491 {
          selector: w491 -> [w496 _]
          tunnel: eventvkey."Left" ("VKey") -> [w494 _]
          frame "Left", "Right" {
            n320 = Equal?(x=w494, y=w496) -> (x = y?=w495:bool)
            n321 = Select(t=0, s=w495, f=1) -> (s? t:f=w497:i32)
            n322 = property on="CheckList" class="LstBox (strict)"() -> ("Item Symbols"=w500:i32[])  [unwired: 2 in, 2 out]
            n323 = Replace Array Subset(array=w500, new element=w497, index="CheckList") -> (w499:i32[])
            n324 = property on="CheckList" class="LstBox (strict)"("Item Symbols"=w499) -> ()  [unwired: 2 in, 2 out]
          }
          frame Default {
          }
        }
      }
      event "Motor.Enable": Value Change {
        # "When the test mode otor enable helper is set, update that\ntree row item's value"
        n325 = event-data() -> ("NewVal"=w506:bool)  [unwired: 1 in]
        n326 = Unbundle("Motor") -> ("Value"=w505:dbl)  [unwired: 1 out]
        n327 = Select(t=w505, s=w506, f=0.0) -> (s? t:f=w503:dbl)
        n328 = call <vilib>:"NT Write Number.vi"("Numeric"=w503, "Name"=w502) -> ()  [unwired: 9 in, 1 out]
      }
      event "Test Slider": Value Change {
        # "When the test mode slider helper is set, update that\ntree row item's value"
        n329 = event-data() -> ("NewVal"=w509:dbl)  [unwired: 1 in]
        n330 = call <vilib>:"NT Write Number.vi"("Numeric"=w509, "Name"=w510) -> ()  [unwired: 9 in, 1 out]
      }
      event "On/Off": Value Change {
        # "When the test mode on/off helper value is set, update that\ntree row item's value"
        n331 = event-data() -> ("NewVal"=w514:bool)  [unwired: 1 in]
        n332 = Boolean To (0,1)(Boolean=w514) -> (0, 1=w513:i16)
        n333 = call <vilib>:"NT Write Number.vi"("Numeric"=w513, "Name"=w512) -> ()  [unwired: 9 in, 1 out]
      }
      event "Rev/Fwd": Value Change {
        # "When the test mode helper value for relays is set, update that\ntree row item's value"
        n334 = event-data() -> ("NewVal.Forward"=w522:bool, "NewVal.Reverse"=w521:bool)  [unwired: 1 in]
        n335 = Boolean To (0,1)(Boolean=w522) -> (0, 1=w518:i16)
        n336 = Boolean To (0,1)(Boolean=w521) -> (0, 1=w520:i16)
        n337 = Negate(x=w520) -> (-x=w519:i16)
        n338 = Add(x=w518, y=w519) -> (x+y=w517:i16)
        n339 = call <vilib>:"NT Write Number.vi"("Numeric"=w517, "Name"=w516) -> ()  [unwired: 9 in, 1 out]
      }
      event "Test Ring": Value Change {
        # "When a test mode helper value is selected from the ring,\nset the tree item's variable to the string value"
        n340 = event-data() -> ("NewVal"=w526:u16)  [unwired: 1 in]
        n341 = property on="Test Ring" class="Ring (strict)"() -> ("Strings []"=w527:string[])  [unwired: 2 in, 2 out]
        n342 = Index Array(array=w527, index=w526) -> (element=w525:string)
        n343 = call <vilib>:"NT Write String.vi"("String"=w525, "Name"=w524) -> ()  [unwired: 9 in, 1 out]
      }
      event "Rec Mode": Value Change {
        # "Update globals for recording mode and path to read log from.\nClear when logging and let NetworkTables set path for vision to\nuse."
        n344 = event-data() -> ("NewVal"=w538:enum32{"Stop", "Record", "Playback"})  [unwired: 1 in]
        n345 = global write "WPI_DashboardLogging Global.vi" "Logging Filename"(path "") -> ()
        n346 = global write "WPI_DashboardLogging Global.vi" "Recording"(w538) -> ()
        n347 = case shown="\"Playback\"" w538 {
          tunnel: w537 -> [_ w540 w549]
          tunnel: [_ _ w548] -> w535
          tunnel: [_ _ w547] -> _
          tunnel: w533 -> [_ _ w545]
          tunnel: cluster{i32, i32} {-250, 170} -> [_ _ w544]
          tunnel: [_ _ T23 {"Image Size"=TRUE, "Image Type"=TRUE, "Pixel Value"=TRUE, "ROI Information"=TRUE, "Zoom Factor"=FALSE} ("Image Information Shown:All Elements")] -> w528
          tunnel: [_ _ TRUE ("Zoom Factor")] -> w529
          tunnel: w531 -> [_ _ w541]
          frame Default {
          }
          frame "Stop", "Record" {
            # "Place Window too"
            n348 = invoke class="VI" method="FP.Close"(reference=w540) -> (reference out=w539:refnum<vi>)  [unwired: 2 in, 2 out]
            n349 = invoke class="VI" method="Abort VI"(reference=w539) -> ()  [unwired: 2 in, 3 out]
          }
          frame "Playback" {
            n350 = call "Open Playback Panel.vi"("Offset"=w544, "DB VI Ref"=w545, "Playback in"=w549) -> ("Playback out"=w546:refnum<vi>)  [unwired: 8 in]
            n351 = register-events(w546, w541) -> (reference out=w548:refnum<event-registration>, error out=w547:errorcluster)  [unwired: 2 in]
          }
        }
        n352 = property on="Camera Image Right" class="ImageControl"("Image Information Shown"=w528, "Image Information Visible"=w529) -> ()  [unwired: 2 in, 2 out]
        n353 = property on="Camera Image" class="ImageControl"("Image Information Shown"=w528, "Image Information Visible"=w529) -> ()  [unwired: 2 in, 2 out]
        n354 = call <vilib>:"WPI_DashboardNT Log FieldName Cache.vi"("Operation"=enum16{"Lookup/Add", "Index", "Clear"}."Clear") -> ()  [unwired: 8 in, 3 out]
      }
      event Panel Close {
        w551 = enum32{"Stop", "Record", "Playback"}."Stop" ("Rec Mode")
        # "Playback window has been closed, abort"
        n355 = event-data() -> ()  [unwired: 1 in, 4 out]
        n356 = local write "Rec Mode"(w551) -> ()
        n357 = global write "WPI_DashboardLogging Global.vi" "Recording"(w551) -> ()
      }
      event Panel Close {
        # "Abort playback window and ourself"
        n358 = event-data() -> ()  [unwired: 1 in, 4 out]
        n359 = invoke class="VI" method="FP.Close"(reference=w555) -> (reference out=w554:refnum<vi>)  [unwired: 2 in, 2 out]
        n360 = invoke class="VI" method="Abort VI"(reference=w554) -> (error out=w553:errorcluster)  [unwired: 2 in, 2 out]
        n361 = invoke class="VI" method="Abort VI"(error in=w553) -> ()  [unwired: 2 in, 3 out]
      }
      event User Event {
        n362 = event-data() -> ("IDs"=w562:cluster{"RPC field ID":u16, "Unique ID":u16}, "String"=w561:string)  [unwired: 1 in]
        n363 = Bundle("IDs"=w562, "String"=w561) -> (w560:T10)  [unwired: 1 in]
        n364 = call <vilib>:"Retrieve RPC Response.vi"("RPC Response"=w560) -> ("Output"=w558:string[][])  [unwired: 10 in]
        n365 = Build Array (concatenate)(w556, w558) -> (w557:string[][])
        n366 = local write "Command Params"(w557) -> ()
        n367 = local write "Cmd Status"("" ("Cmd Status")) -> ()
      }
      event "Tree": Double Click {
        n368 = event-data() -> ("PlatMods"=w568:T26, "Tag"=w565:string)  [unwired: 1 in]
        n369 = Unbundle(w568) -> ("Shift"=w567:bool)  [unwired: 4 out]
        n370 = String Subset(string=w565, length (rest)=1 ("length (rest)")) -> (substring=w564:string)  [unwired: 1 in]
        n371 = Not(x=w567) -> (.not. x?=w566:bool)
        n372 = case shown="\"/\"" w564 {
          tunnel: w565 -> [_ w571]
          tunnel: w566 -> [_ w570]
          frame Default {
          }
          frame "/" {
            n373 = call <vilib>:"NT Update Persistence.vi"("Persistence"=w570, "Name"=w571) -> ()  [unwired: 9 in, 1 out]
          }
        }
      }
    }
  }
  n374 = while {
    tunnel: w65 -> [w573]
    i -> [w576]
    stop <- FALSE stop-if-true
    n375 = Wait (ms)(milliseconds to wait=u32 100) -> ()  [unwired: 1 out]
    n376 = case shown="\"Playback\"" "Rec Mode" {
      tunnel: w576 -> [_ _ w591]
      tunnel: [u32 2829099 ("Base Color") u32 11141120 ("Target Color") w580] -> w572
      frame "Stop", Default {
        # "Reset the color, extra updates don't cost much"
      }
      frame "Record" {
      }
      frame "Playback" {
        # "Playback"
        n377 = Quotient & Remainder(x=w591, y=u32 50 ("milliseconds to wait")) -> (x-y*floor(x/y)=w587:u32)  [unwired: 1 out]
        n378 = Divide(x=w587, y=u32 50 ("milliseconds to wait")) -> (x/y=w584:dbl)
        n379 = Multiply(x=6.283185307179586, y=w584) -> (x*y=w589:dbl)
        n380 = Sine(x=w589) -> (sin(x)=w588:dbl)
        n381 = Absolute Value(x=w588) -> (abs(x)=w581:dbl)
        n382 = call "Interpolate RGB Color.vi"("Proportion"=w581, "Target Color"=u32 30976, "Base Color"=u32 2829099) -> ("Result Color"=w580:u32)  [unwired: 8 in]
      }
    }
    n383 = property class="Pane"(reference=w573, "PaneColor"=w572) -> ()  [unwired: 1 in, 2 out]
  }
  n384 = local write "Dashboard Tab"(T2."Drive" ("Dashboard Tab")) -> ()
  n385 = property on="On/Off" class="Bool (strict)"("Visible"=w36) -> ()  [unwired: 2 in, 2 out]
  n386 = property on="Motor" class="Clust (strict)"("Visible"=w36) -> ()  [unwired: 2 in, 2 out]
  n387 = property on="Progress" class="Clust (strict)"("Visible"=w36) -> ()  [unwired: 2 in, 2 out]
  n388 = property on="Test Ring" class="Ring (strict)"("Visible"=w36) -> ()  [unwired: 2 in, 2 out]
  n389 = property on="Rev/Fwd" class="Clust (strict)"("Visible"=w36) -> ()  [unwired: 2 in, 2 out]
  n390 = local write "Command Selection"(u16 0 ("milliseconds to wait")) -> ()
  n391 = while {
    tunnel: u16 1741 ("timeout ms (25000)") -> [w593]
    stop <- FALSE stop-if-true
    n392 = TCP Create Listener(10:w593) -> (0:w592:errorcluster, 3:w594:refnum<k5>)  [unwired: 4 in, 1 out]
    n393 = case shown="No Error" w592 {
      selector: w592 -> [w596 _]
      tunnel: w594 -> [w597 _]
      frame No Error {
        n394 = while {
          tunnel: w597 -> [w600]
          tunnel: w596 -> [w599]
          stop <- FALSE stop-if-true
          n395 = TCP Wait On Listener(8:w599, 11:w600) -> (0:w601:errorcluster, 4:w602:refnum<k5>)  [unwired: 2 in, 3 out]
          n396 = local write "TCP"(w602) -> ()
          n397 = case shown="No Error" w601 {
            frame No Error {
            }
            frame Error {
              n398 = Wait (ms)(milliseconds to wait=u32 1000) -> ()  [unwired: 1 out]
            }
          }
        }
      }
      frame Error {
        n399 = Wait (ms)(milliseconds to wait=u32 1000) -> ()  [unwired: 1 out]
      }
    }
  }
  n400 = local write "Command Params"(string[][] [] ("Command Params")) -> ()
  n401 = global write "WPI_DashboardLogging Global.vi" "Recording"(w59) -> ()
  n402 = local write "Rec Mode"(w59) -> ()
  n403 = call <vilib>:"NT Write String.vi"("String"="Select Auto", "Name"="Auto Selector") -> ()  [unwired: 9 in, 1 out]
